vi "get severity.vi"(11 "exception in":T2 {"code" format="%.0x"}) -> (2 "severity":T1, 3 "exception out":T2 {"code" format="%.0x"})   [LabVIEW 2013, in "exception.lvlib"]
uses:
  exception.lvlib
  exception.ctl
  severity.ctl
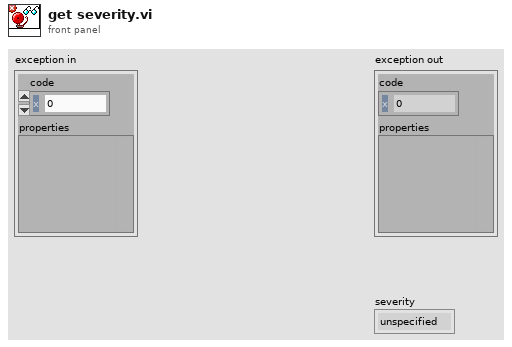
[diagram p1: front panel]
types:
  T1 = typedef "exception.lvlib/severity.ctl" = enum8{"unspecified", "informational", "operation failed", "data corruption", "system corruption", "critical unknown state"}
  T2 = typedef "exception.lvlib/exception.ctl" = cluster{"code":i32, "properties":variant}
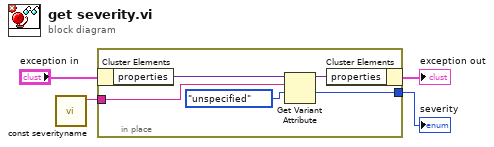
[diagram p0: block diagram]
diagram:
  n1 = call "const severityname.vi"() -> ("label"=w2:string)  [unwired: 11 in]
  n2 = in-place {
    in-place-border: w2 -> [w7]
    in-place-border: [w6] -> w1
    n3 = in-place-cluster #1("exception in") -> ("properties"=w9:variant)
    n4 = Get Variant Attribute(Variant=w9, name=w7, default value (empty Variant)=severity."unspecified" ("severity")) -> (duplicate Variant=w8:variant, value=w6:T1)  [unwired: 1 in, 2 out]
    n5 = in-place-cluster #1("properties"=w8) -> (→"exception out":T2)
  }
  "severity" <- w1
